vi "Full Example.vi"() -> ()   [LabVIEW 2020, in "Tests.lvlib"]
uses:
  4256cc0c-174c-4abd-a533-76f0a5263063.vi
  f430c4b3-d20c-4940-9a34-8d4ef63f415b.vi
  7957bec0-3d3d-4ed0-aecb-9f5c57c08ef2.vi
  19ea942b-b215-4be2-9d4a-2ca72531a5b1.vi
  b560e9f3-cc2a-438b-800e-d8071980c137.vi
  dc2271b3-c93b-4ea0-963d-17d3fd46d2d4.vi
  73432ad2-7848-4561-9f03-722614b77e3c.vi
  19ea942b-b215-4be2-9d4a-2ca72531a5b1.vi/35c0bed4-0107-49e5-a1be-c3402b1a4269.vi
  19ea942b-b215-4be2-9d4a-2ca72531a5b1.vi/4b1c2d87-9503-4854-8dc7-31bb0771dd1b.vi
  b560e9f3-cc2a-438b-800e-d8071980c137.vi/35c0bed4-0107-49e5-a1be-c3402b1a4269.vi
  b560e9f3-cc2a-438b-800e-d8071980c137.vi/4b1c2d87-9503-4854-8dc7-31bb0771dd1b.vi
  b560e9f3-cc2a-438b-800e-d8071980c137.vi/4049b438-30ac-40ac-bf8b-38a25aeeaacb.vi
  dc2271b3-c93b-4ea0-963d-17d3fd46d2d4.vi/6603e637-5b00-4c85-831f-438498c6f5cd.vi
  dc2271b3-c93b-4ea0-963d-17d3fd46d2d4.vi/435e0bdd-08e9-4973-aa49-bb73efdc2477.vi
  <vilib>/dlg_ctls.llb/Space Constant.vi
  dc2271b3-c93b-4ea0-963d-17d3fd46d2d4.vi/b24c019a-0099-4d06-9010-75d0c3ff117b.vi
  73432ad2-7848-4561-9f03-722614b77e3c.vi/6603e637-5b00-4c85-831f-438498c6f5cd.vi
  73432ad2-7848-4561-9f03-722614b77e3c.vi/435e0bdd-08e9-4973-aa49-bb73efdc2477.vi
  73432ad2-7848-4561-9f03-722614b77e3c.vi/48c7ac7e-bb0d-49e2-af2c-796dbdcbcaf5.vi
  dc2271b3-c93b-4ea0-963d-17d3fd46d2d4.vi/6603e637-5b00-4c85-831f-438498c6f5cd.vi/35c0bed4-0107-49e5-a1be-c3402b1a4269.vi
  dc2271b3-c93b-4ea0-963d-17d3fd46d2d4.vi/6603e637-5b00-4c85-831f-438498c6f5cd.vi/4b1c2d87-9503-4854-8dc7-31bb0771dd1b.vi
  dc2271b3-c93b-4ea0-963d-17d3fd46d2d4.vi/435e0bdd-08e9-4973-aa49-bb73efdc2477.vi/35c0bed4-0107-49e5-a1be-c3402b1a4269.vi
  dc2271b3-c93b-4ea0-963d-17d3fd46d2d4.vi/435e0bdd-08e9-4973-aa49-bb73efdc2477.vi/4b1c2d87-9503-4854-8dc7-31bb0771dd1b.vi
  dc2271b3-c93b-4ea0-963d-17d3fd46d2d4.vi/435e0bdd-08e9-4973-aa49-bb73efdc2477.vi/4049b438-30ac-40ac-bf8b-38a25aeeaacb.vi
  73432ad2-7848-4561-9f03-722614b77e3c.vi/6603e637-5b00-4c85-831f-438498c6f5cd.vi/35c0bed4-0107-49e5-a1be-c3402b1a4269.vi
  73432ad2-7848-4561-9f03-722614b77e3c.vi/6603e637-5b00-4c85-831f-438498c6f5cd.vi/4b1c2d87-9503-4854-8dc7-31bb0771dd1b.vi
  73432ad2-7848-4561-9f03-722614b77e3c.vi/435e0bdd-08e9-4973-aa49-bb73efdc2477.vi/35c0bed4-0107-49e5-a1be-c3402b1a4269.vi
  73432ad2-7848-4561-9f03-722614b77e3c.vi/435e0bdd-08e9-4973-aa49-bb73efdc2477.vi/4b1c2d87-9503-4854-8dc7-31bb0771dd1b.vi
  73432ad2-7848-4561-9f03-722614b77e3c.vi/435e0bdd-08e9-4973-aa49-bb73efdc2477.vi/4049b438-30ac-40ac-bf8b-38a25aeeaacb.vi
  Examples/Capitalize.vi
  Examples/Is Even.vi
  Tests.lvlib
  Examples/Examples.lvlib
panel:
  out "Final String":string
  in  "Strings":string[](array[string])=["[Person]", "first-name = Jim", "last-name = Bob", "age = 31"]
  out "Even Numbers":i32[](array[numeric])
  in  "Numbers":i32[](array[numeric])=[-3, -2, -1, 0, 1, 2, 3, 4, 5]
  out "Capitalized Strings":string[](array[string])
  in  "Strings":string[](array[string])=["test", "string", "word"]
  out "D":u16[](array[numeric])
  out "C":dbl[](array[numeric]) format="%.2f"
  out "B":i32[](array[numeric])
  out "A":dbl[](array[numeric]) format="%.2f"
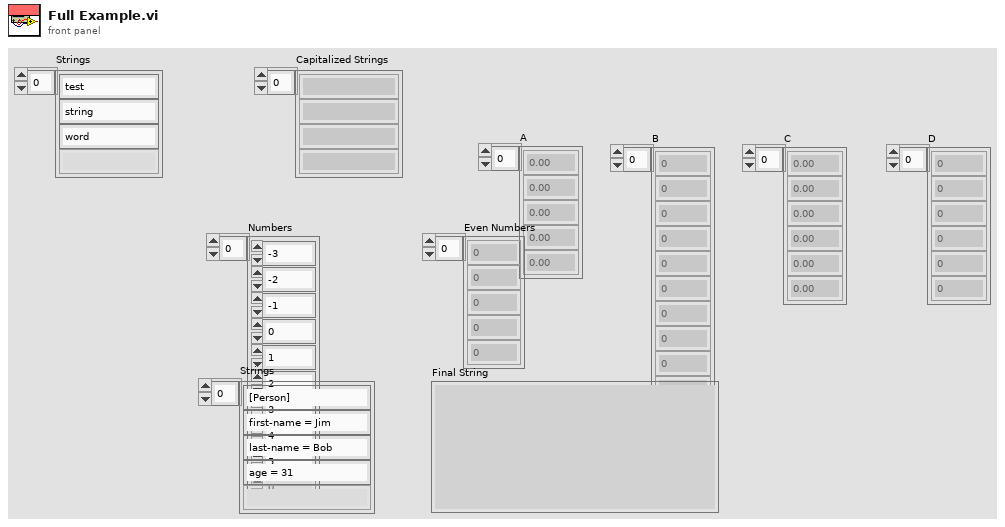
[diagram p1: front panel]
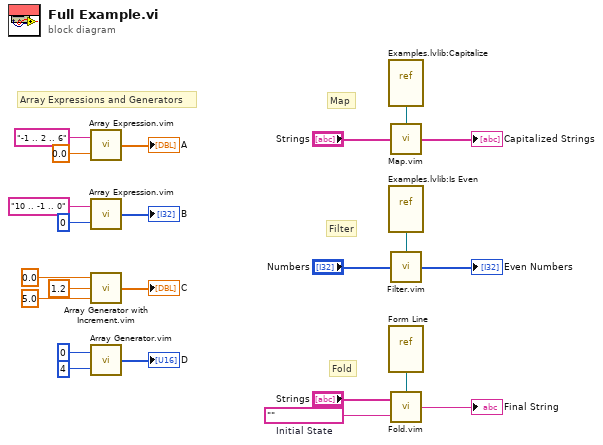
[diagram p0: block diagram]
diagram:
  w3 = ""  # Initial State
  # "Array Expressions and Generators"
  # "Fold"
  # "Filter"
  # "Map"
  n1 = call "Array Expression.vim"("Type"=0.0, "Expression"="-1 .. 2 .. 6") -> ("Array"=→"A":dbl[])
  n2 = call "Array Expression.vim"("Type"=0, "Expression"="10 .. -1 .. 0") -> ("Array"=→"B":i32[])
  n3 = call "Array Generator with Increment.vim"("Until"=5.0, "Increment"=1.2, "Begin"=0.0) -> ("Array"=→"C":dbl[])
  n4 = call "Array Generator.vim"("End"=u16 4, "Begin"=u16 0) -> ("Array"=→"D":u16[])
  n5 = vi-ref "Examples.lvlib:Capitalize.vi"() -> (w10:refnum<vi>)
  n6 = vi-ref "Examples.lvlib:Is Even.vi"() -> (w7:refnum<vi>)
  n7 = vi-ref "Form Line.vi"() -> (w4:refnum<vi>)
  n8 = call "Map.vim"("Processor"=w10, "Array"="Strings") -> ("Mapped Array"=→"Capitalized Strings":string[])  [unwired: 2 in]
  n9 = call "Filter.vim"("Predicate"=w7, "Array"="Numbers") -> ("Filtered Array"=→"Even Numbers":i32[])  [unwired: 2 in]
  n10 = call "Fold.vim"("Processor"=w4, "Initial State"=w3, "Array"="Strings") -> ("Final State"=→"Final String":string)
